vi "HHMI - Count U32 with saturate.vi"(7 "Reset?":bool, 10 "Increment?":bool) -> (2 "total # counted\n(Reset occurs \nprior to Increment)":u32)   [LabVIEW 2013]
doc: "Counts up. Reset returns count to zero. Increment occurs after Reset."
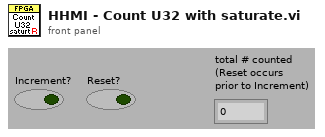
[diagram p1: front panel]
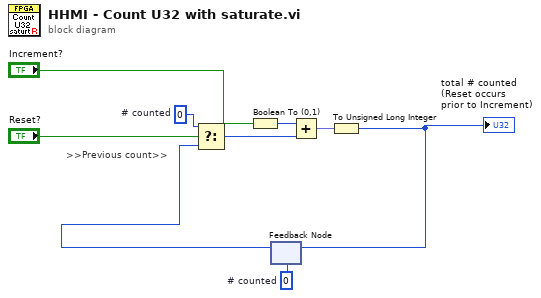
[diagram p0: block diagram]
diagram:
  w6 = u32 0  # # counted
  w9 = u32 0  # # counted
  # ">>Previous count>>"
  n1 = Boolean To (0,1)(Boolean="Increment?") -> (0, 1=w5:i16)
  n2 = feedback #1(w9) -> (w7:u32)
  n3 = Select(t=w6, s="Reset?", f=w7) -> (s? t:f=w3:u32)
  n4 = Add(x=w5, y=w3) -> (x+y=w2:fxp<+,32,32>)
  n5 = To Unsigned Long Integer(number=w2) -> (unsigned 32bit integer=w1:u32)
  "total # counted\n(Reset occurs \nprior to Increment)" <- w1
  n6 = feedback-in #1(w1) -> ()
